vi "Open API Tester.vi"(11 "Event vi Ref":refnum<vi>) -> (0 "error out":errorcluster)   [LabVIEW 2020, in "Panther Dashboard.lvlib"]
doc: "This VI checks the Main.vi State of the selected DQMH Module"
uses:
  Panther Dashboard.lvlib
panel:
  in  "error in (no error)":errorcluster
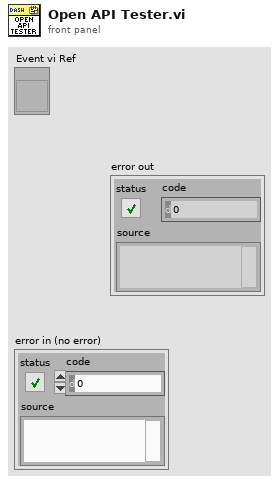
[diagram p1: front panel]
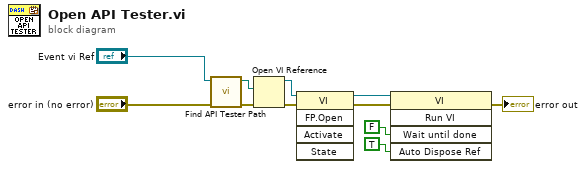
[diagram p0: block diagram]
diagram:
  n1 = call "Find API Tester Path.vi"("error in"="error in (no error)", "Event vi Ref"="Event vi Ref") -> ("error out"=w7:errorcluster, "API Tester Path"=w2:path)  [unwired: 8 in]
  n2 = Open VI Reference(vi path=w2, error in (no error)=w7) -> (vi reference=w6:refnum<vi>, error out=w11:errorcluster)  [unwired: 4 in]
  n3 = invoke class="VI" method="FP.Open"(reference=w6, error in=w11) -> (reference out=w5:refnum<vi>, error out=w10:errorcluster)  [unwired: 3 in, 3 out]
  n4 = invoke class="VI" method="Run VI"(reference=w5, error in=w10, "Wait until done"=FALSE ("Wait Until Done"), "Auto Dispose Ref"=TRUE ("Auto Dispose Reference")) -> (error out=→"error out":errorcluster)  [unwired: 1 in, 4 out]
